vi "Init Sound Card.vi"() -> (0 "error out":errorcluster, 1 "task ID":T1 format="%.0x")   [LabVIEW 2011, in "LabVIEW Interface for ChipKit.lvlib"]
uses:
  LabVIEW Interface for ChipKit.lvlib
  <vilib>/sound2/lvsound2.llb/Sound Output Task ID.ctl
  <vilib>/sound2/lvsound2.llb/Sampling Mode.ctl
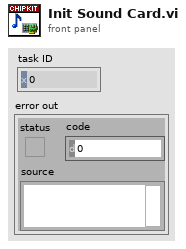
[diagram p1: front panel]
types:
  T1 = typedef "Sound Output Task ID.ctl" = u32
  T2 = typedef "Sampling Mode.ctl" = i32
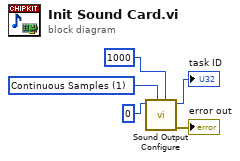
[diagram p0: block diagram]
diagram:
  w3 = T2 1 items=["Finite Samples", "Continuous Samples"] ("sample mode")
  n1 = call <vilib>:"Sound Output Configure.vi"("number of samples/ch"=1000, "sample mode"=w3, "device ID"=u32 0) -> ("error out"=→"error out":errorcluster, "task ID"=→"task ID":T1)  [unwired: 7 in]
